vi "Start Instrument Calibration.vi"(8 "error in (no error)":errorcluster, 11 "Instrument Handler in":refnum<class "Instrument Handler.lvclass">) -> (0 "error out":errorcluster, 3 "Instrument Handler out":refnum<class "Instrument Handler.lvclass">)   [LabVIEW 2020, in "Instrument Handler.lvlib" / "Instrument Handler.lvclass"]
doc: "Get all launched instruments and start calibration of these instruments."
uses:
  Instrument Handler.lvclass
  C:/Current projects/WS/PPL/HDH.Actor Framework.Core.Actor.lvlibp/1abvi3w/vi.lib/ActorFramework/Actor/Actor.lvclass
  Controls/Ctl_InstrumentSynchronicationCluster.ctl
  PPL/HDH.Actor Framework.Core.Instrument Driver.lvlibp/Instrument Driver/Controls/Ctl_ConnectionType.ctl
  PPL/HDH.Data.Generic.lvlibp/Synchronization/Notifier/Notifier.lvclass
  PPL/HDH.Actor Framework.Core.Actor.lvlibp/1abvi3w/vi.lib/ActorFramework/Message Enqueuer/Message Enqueuer.lvclass
  PPL/HDH.Actor Framework.Core.Sequencer.lvlibp/Sequencer Core/Sequencer Core.lvclass
  Messages/Calibrate Instrument Msg/Calibrate Instrument Msg.lvclass
  C:/Current projects/WS/PPL/HDH.Actor Framework.Core.Publisher.lvlibp/Messages/Response Msg/Response Msg.lvclass
  PPL/HDH.Actor Framework.Core.Publisher.lvlibp/Messages/Response Msg/Response Core/Controls/Ctl_SendFunction.ctl
  Instrument Handler.lvclass/Instrument Handler.ctl
  PPL/HDH.Actor Framework.Core.Publisher.lvlibp/Publisher Messages/Bypass Msg/Bypass Msg.lvclass
  C:/Current projects/WS/PPL/HDH.Actor Framework.Core.Publisher.lvlibp/Publisher Messages/Sender Msg/Sender Msg.lvclass
  PPL/HDH.Actor Framework.Core.Instrument Driver.lvlibp/Instrument Driver/Instrument Driver.lvclass
  Instrument Handler.lvlib
  PPL/HDH.Actor Framework.Core.Publisher.lvlibp/Messages/Response Msg/Response Msg.lvclass
  PPL/HDH.Actor Framework.Core.Publisher.lvlibp
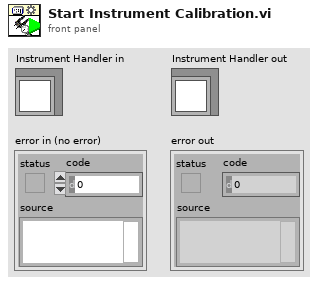
[diagram p1: front panel]
types:
  T1 = typedef "HDH.Actor Framework.Core.Publisher.lvlibp/Ctl_SendFunction.ctl" = enum16{"Send and Forget", "Request Reply", "Await Reply"}
  T2 = typedef "Instrument Handler.lvlib/Ctl_InstrumentSynchronicationCluster.ctl" = cluster{"Launched?":bool, "Driver Path":path, "Alias":string, "Connection Type":T3, "Pre Initialization Data":variant, "Enqueue Sync":refnum<class "Notifier.lvclass">, "Enqueue Lock":T4, "Owner Enqueuer":refnum<class "Message Enqueuer.lvclass">, "Owner":refnum<class "Sequencer Core.lvclass">, "Instrument ID":u32}
  T3 = typedef "HDH.Actor Framework.Core.Instrument Driver.lvlibp/Instrument Driver.lvclass/Ctl_ConnectionType.ctl" = enum16{"BuiltIn/System", "PXI/PCI", "USB", "GPIB", "VXI", "Serial", "TCP/IP", "cRIO", "SCXI", "cDAQ", "SwitchBlock", "SCC", "FireWire", "Accessory", "CAN", "SwitchBlock Device"}
  T4 = typedef "Semaphore RefNum" = refnum<k1>
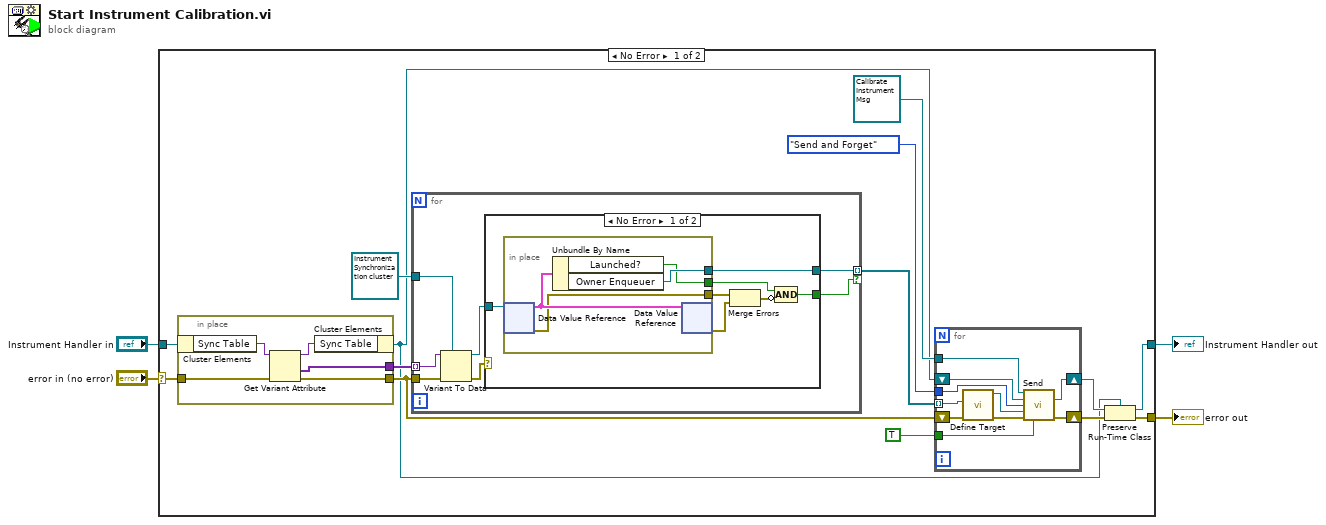
[diagram p0: block diagram]
diagram:
  n1 = case shown="No Error" "error in (no error)" {
    selector: "error in (no error)" -> [w15 w53]
    tunnel: [w9 w53] -> w3
    tunnel: [w7 w52] -> w1
    tunnel: "Instrument Handler in" -> [w18 w52]
    frame No Error {
      n2 = in-place {
        in-place-border: [w49] -> w17
        in-place-border: w15 -> [w48]
        in-place-border: [w47] -> w11
        n3 = in-place-cluster #1(w18) -> ("Sync Table"=w51:variant)
        n4 = Get Variant Attribute(Variant=w51, error in=w48) -> (duplicate Variant=w50:variant, values=w49:variant[], error out=w47:errorcluster)  [unwired: 2 in, 1 out]
        n5 = in-place-cluster #1("Sync Table"=w50) -> (w6:refnum<class "Instrument Handler.lvclass">)
      }
      n6 = for {
        tunnel: w17 -> [w35] mode=indexing
        tunnel: refnum<data-value> refnum ("data value reference") -> [w34]
        tunnel: w11 -> [w31]
        tunnel: [w30] -> w5 mode=indexing if=w29
        n7 = Variant To Data(error in=w31, type=w34, Variant=w35) -> (data=w32:refnum<data-value>, error out=w33:errorcluster)
        n8 = case shown="No Error" w33 {
          tunnel: w32 -> [w42 _]
          tunnel: [w41 _] -> w30
          tunnel: [w38 _] -> w29
          frame No Error {
            n9 = in-place {
              in-place-border: [w45] -> w41
              in-place-border: [w44] -> w37
              in-place-border: [w43] -> w40
              n10 = in-place-dvr #2(w42) -> (w46:T2, w43:errorcluster)
              n11 = Unbundle By Name(w46) -> ("Launched?"=w44:bool, "Owner Enqueuer"=w45:refnum<class "Message Enqueuer.lvclass">)
              n12 = in-place-dvr #2(w46) -> (w39:errorcluster)  [unwired: 1 out]
            }
            n13 = Merge Errors(w40, w39) -> (w36:errorcluster)
            n14 = Compound Arithmetic op=AND(w37, invert w36) -> (w38:bool)
          }
          frame Error {
          }
        }
      }
      n15 = for {
        tunnel: Ctl_SendFunction."Send and Forget" ("Send Function") -> [w28]
        tunnel: TRUE ("Publish Data?(F)") -> [w27]
        tunnel: refnum<class "Calibrate Instrument Msg.lvclass"> refnum ("Instrument Handler.lvlib:Calibrate Instrument Msg.lvclass") -> [w26]
        shift-right: [w22] -> w10
        shift-left: w11 -> [w24]
        shift-right: [w21] -> w8
        shift-left: w6 -> [w20]
        tunnel: w5 -> [w19] mode=indexing
        n16 = call "Define Target.vi"("error in (no error)"=w24, "Target Enqueuer"=w19) -> ("error out"=w23:errorcluster, "Targetted Msg out"=w25:refnum<class "Bypass Msg.lvclass">)  [unwired: 8 in]
        n17 = call "Send.vi"("Response Msg in"=w26, "Actor in"=w20, "Send Function"=w28, "Sender (publish)"=w25, "error in (no error)"=w23, "Publish Data?(F)"=w27) -> ("Actor out"=w21:refnum<class "Actor.lvclass">, "error out"=w22:errorcluster)  [unwired: 5 in, 3 out]
      }
      n18 = Preserve Run-Time Class(object in=w8, error in=w10, 2:w6) -> (object out=w7:refnum<class "Instrument Handler.lvclass">, error out=w9:errorcluster)
    }
    frame Error {
    }
  }
  "error out" <- w3
  "Instrument Handler out" <- w1
